vi "Simple UDP - Sender2.vi"() -> ()   [LabVIEW 2013]
doc: "The UDP protocol differs from TCP in that there is no error-checking with the packets of information that are sent, and thus no guarantee whatsoever that an intended recipient will actually receive a given piece of data.\n\nUDP does offer the ability to \"broadcast\" data across a network--simply specify an IP Address of all ones (255.255.255.255) to attempt to broadcast information network-wide. Keep in mind that routers and other network hardware will generally refuse to forward the broadcast beyond certain points, so the extent of the broadcast will in practice be limited."
panel:
  out "Current Data Value":dbl
  in  "Stop":bool
  # "Overview: Demonstrates the use of the UDP functions to send data over a UDP connection.\nInstructions:\n1. Run the VI.\n2. Open Simple UDP - Receiver.vi and follow the instructions on its front panel.\n3. Click Stop to stop the VI."
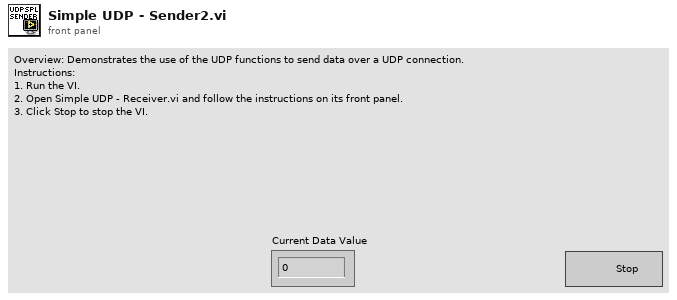
[diagram p1: front panel]
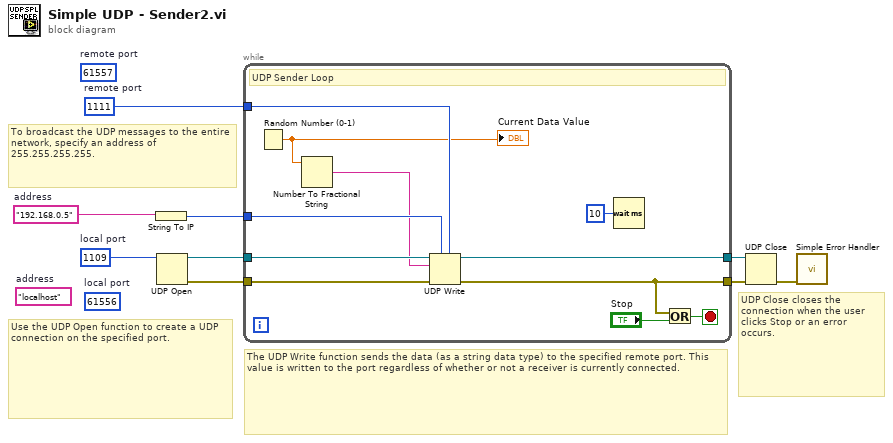
[diagram p0: block diagram]
diagram:
  (unwired) u16 61557  # remote port
  (unwired) u16 61556  # local port
  w1 = "192.168.0.5"  # address
  w2 = u16 1111  # remote port
  w3 = u16 1109  # local port
  (unwired) "localhost"  # address
  # "To broadcast the UDP messages to the entire network, specify an address of 255.255.255.255."
  # "UDP Close closes the connection when the user clicks Stop or an error occurs."
  # "The UDP Write function sends the data (as a string data type) to the specified remote port. This value is written to the port regardless of whether or not a receiver is currently connected."
  # "Use the UDP Open function to create a UDP connection on the specified port."
  n1 = String To IP(1:w1) -> (0:w6:u32)
  n2 = UDP Open(11:w3) -> (port=w5:refnum<k16>, 0:w4:errorcluster)  [unwired: 4 in, 1 out]
  n3 = while {
    tunnel: [w15] -> w8
    tunnel: w5 -> [w20]
    tunnel: w4 -> [w19]
    tunnel: [w16] -> w9
    tunnel: w6 -> [w14]
    tunnel: w2 -> [w11]
    stop <- w18 stop-if-true
    # "UDP Sender Loop"
    n4 = Random Number (0-1)() -> (number: 0 to 1=w10:dbl)
    "Current Data Value" <- w10
    n5 = Number To Fractional String(number=w10) -> (F-format string=w12:string)  [unwired: 3 in]
    n6 = UDP Write(address=w14, port or service name=w11, connection ID=w20, data in=w12, 8:w19) -> (error out=w15:errorcluster, 3:w16:refnum<k16>)  [unwired: 1 in]
    n7 = Wait (ms)(milliseconds to wait=u32 10) -> ()  [unwired: 1 out]
    n8 = Or(x=w15, y="Stop") -> (x .or. y?=w18:bool)
  }
  n9 = UDP Close(connection ID=w9, 8:w8) -> (error out=w7:errorcluster)  [unwired: 1 out]
  n10 = call <vilib>:"Simple Error Handler.vi"("error in (no error)"=w7) -> ()  [unwired: 4 in, 5 out]
